vi "FPParseLeidenComputerNames.vi"(8 "error in (no error)":errorcluster, 10 "computer name":string="custardpie") -> (0 "error out":errorcluster, 2 "FP Type":enum32{"CF", "Wet"}(ring))   [LabVIEW 2013]
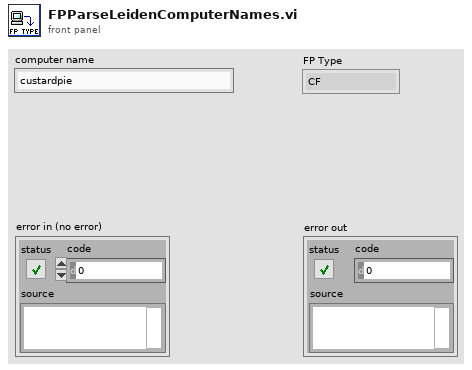
[diagram p1: front panel]
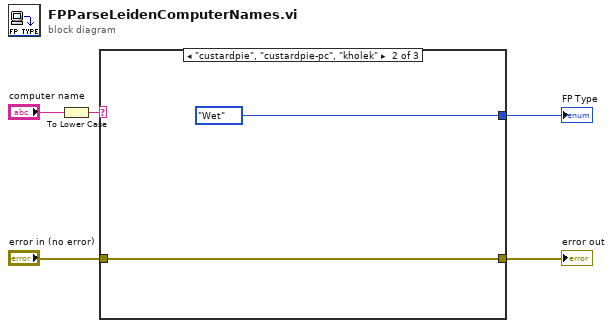
[diagram p0: block diagram]
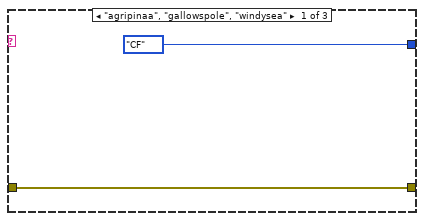
[diagram p2: hidden frame]
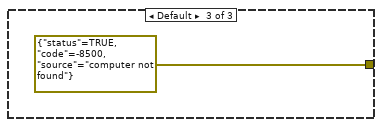
[diagram p3: hidden frame]
diagram:
  n1 = To Lower Case(string="computer name") -> (all lower case string=w1:string)
  n2 = case shown="\"custardpie\", \"custardpie-pc\", \"kholek\"" w1 {
    tunnel: [enum32{"CF", "Wet"}."CF" ("Type") enum32{"CF", "Wet"}."Wet" ("Type") _] -> w5
    tunnel: "error in (no error)" -> [w6 w8 _]
    tunnel: [w6 w8 errorcluster {"status"=TRUE, "code"=-8500, "source"="computer not found"} ("error in (no error)")] -> w2
    frame "agripinaa", "gallowspole", "windysea" {
    }
    frame "custardpie", "custardpie-pc", "kholek" {
    }
    frame Default {
    }
  }
  "FP Type" <- w5
  "error out" <- w2
